vi "main.vi"() -> ()   [LabVIEW 2023]
uses:
  combination.vi
panel:
  out "ans2":i32[](array[numeric])
  out "ans1":i32[](array[numeric])
  in  "limit":i32
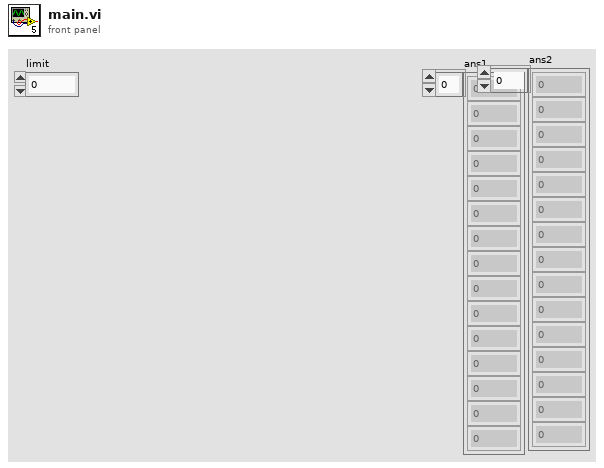
[diagram p1: front panel]
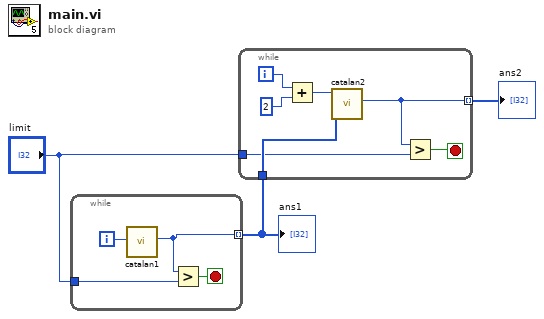
[diagram p0: block diagram]
diagram:
  n1 = while {
    tunnel: "limit" -> [w6]
    tunnel: [w4] -> w3 mode=indexing
    i -> [w5]
    stop <- w7 stop-if-true
    n2 = call "catalan1.vi"("n"=w5) -> ("ans"=w4:i32)  [unwired: 10 in]
    n3 = Greater?(x=w4, y=w6) -> (0:w7:bool)
  }
  "ans1" <- w3
  n4 = while {
    tunnel: w3 -> [w10]
    tunnel: [w9] -> w2 mode=indexing
    tunnel: "limit" -> [w8]
    i -> [w13]
    stop <- w14 stop-if-true
    n5 = Add(x=w13, y=2) -> (x+y=w11:i32)
    n6 = call "catalan2.vi"("past"=w10, "n"=w11) -> ("ans"=w9:i32)  [unwired: 9 in]
    n7 = Greater?(x=w9, y=w8) -> (0:w14:bool)
  }
  "ans2" <- w2
